vi "Do Action.vi"(8 "error in (no error)":errorcluster, 9 "Display Queue":refnum<queue>, 10 "tlc_User Event Reference.ctl":T1, 11 "Exit App in":refnum<class "Exit App.lvclass">) -> (0 "error out":errorcluster)   [LabVIEW 2010, in "Exit App.lvclass"]
doc: "This instance of Do Action.vi is used to perform the functionality that was previously contained in the Exit case of the consumer loop. This method calls tlc_Shutdown.vi to gracefully exit the application when either an error occurs or the user clicks on File»Exit."
uses:
  Exit App.lvclass
  Controls/tlc_User Interface Command.ctl
  Controls/tlc_User Interface Data Type.ctl
  Controls/tlc_User Event Reference.ctl
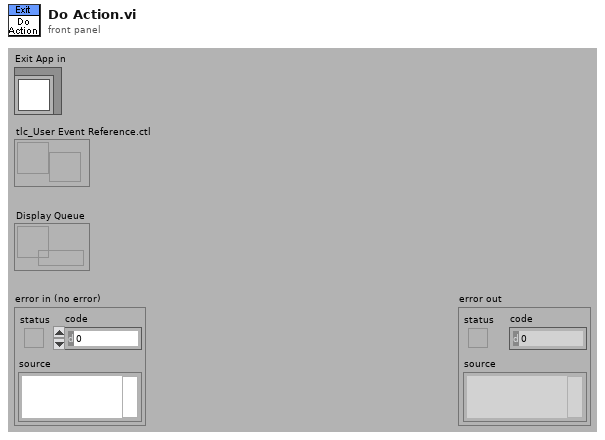
[diagram p1: front panel]
types:
  T1 = typedef "tlc_User Event Reference.ctl" = refnum<user-event>
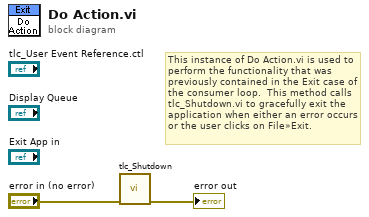
[diagram p0: block diagram]
diagram:
  # "This instance of Do Action.vi is used to \nperform the functionality that was \npreviously contained in the Exit case of \nthe consumer loop.  This method calls \ntlc_Shutdown.vi to gracefully exit the \napplication when either an error occurs \nor the user clicks on File»Exit."
  n1 = call "tlc_Shutdown.vi"("error in (no error)"="error in (no error)") -> ("error out"=→"error out":errorcluster)  [unwired: 10 in]
